vi "FGV_OEE_SQL_connection.vi"(7 "options":T4, 8 "error_in":errorcluster, 9 "all_config_info_in":T1={"main_ini_file"={"SQL Driver"="", "SQL Server"="", "SQL Database"="", "SQL UID"="", "Reference table"="", "Reference history"="", "Archivisation CFG table"="", "Archivisation CFG history"="", "User table"="", "User history"="", "Default reference"="", "Update pulse[ms]"=0, "default language"="", "SCREEN 1 Left"=10, "SCREEN 1 Top"=0, "SCREEN 1 Width"=0, "SCREEN 1 Height"=0, "SCREEN 2 Left"=0, "SCREEN 2 Top"=0, "SCREEN 2 Width"=0, "SCREEN 2 Height"=10}, "SQL Password"="", "queue_refnums"={"MAIN_queue"=refnum, "SCREEN_1_queue"=refnum, "SCREEN_2_queue"=refnum, "PULSE_queue"=refnum, "GRAPH_TOGGLE_queue"=refnum}}, 10 "SQL_transaction":string[](array[string]), 11 "SQL_statement":string) -> (0 "error_out":errorcluster, 1 "all_config_info_out":T1={"main_ini_file"={"SQL Driver"="", "SQL Server"="", "SQL Database"="", "SQL UID"="", "Reference table"="", "Reference history"="", "Archivisation CFG table"="", "Archivisation CFG history"="", "User table"="", "User history"="", "Default reference"="", "Update pulse[ms]"=0, "default language"="", "SCREEN 1 Left"=10, "SCREEN 1 Top"=0, "SCREEN 1 Width"=0, "SCREEN 1 Height"=0, "SCREEN 2 Left"=0, "SCREEN 2 Top"=0, "SCREEN 2 Width"=0, "SCREEN 2 Height"=10}, "SQL Password"="", "queue_refnums"={"MAIN_queue"=refnum, "SCREEN_1_queue"=refnum, "SCREEN_2_queue"=refnum, "PULSE_queue"=refnum, "GRAPH_TOGGLE_queue"=refnum}}, 2 "connection_active?":bool, 3 "SQL_result":variant, 4 "executed_SQL_statement":string)   [LabVIEW 2019]
uses:
  FGV_OEE_SQL_connection.ctl
  ini/typedef/OEE_all_config_info.ctl
  ini/typedef/OEE_main_ini_file.ctl
  queues/typedef/OEE_queue_refnums.ctl
  queues/typedef/OEE_MAIN_queue_element.ctl
  MAIN/OEE_MAIN_sequence_state.ctl
  queues/typedef/OEE_SCREEN_1_queue_element.ctl
  SCREEN_1/OEE_SCREEN_1_sequence_state.ctl
  queues/typedef/OEE_SCREEN_2_queue_element.ctl
  SCREEN_2/OEE_SCREEN_2_sequence_state.ctl
  queues/typedef/OEE_PULSE_queue_element.ctl
  PULSE/OEE_PULSE_sequence_state.ctl
  queues/typedef/OEE_GRAPH_TOGGLE_TIMER_queue_element.ctl
  SCREEN_2/GRAPH_TOGGLE_TIMER/OEE_GRAPH_TOGGLE_TIMER_sequence_state.ctl
  <vilib>/addons/database/Auxilliary.llb/DB Tools Transaction.ctl
  <vilib>/addons/database/Connection.llb/Conn ObjectReference.ctl
  <vilib>/addons/database/Connection.llb/DB Tools Open Connec (String).vi
  <vilib>/addons/database/Connection.llb/Conn Execute.vi
  <vilib>/addons/database/Recordset.llb/Rec Destroy - Connection.vi
  <userlib>/_OpenG.lib/array/array.llb/Filter 1D Array (String)__ogtk.vi
  <vilib>/addons/database/Recordset.llb/Rec Fetch Recordset Data (R).vi
  <vilib>/addons/database/Recordset.llb/Rec Get Recordset Properties (R).vi
  <vilib>/addons/database/Recordset.llb/Rec Get Column Properties (R).vi
  <vilib>/addons/database/Connection.llb/Conn Transaction.vi
  <vilib>/addons/database/NI_Database_API.lvlib
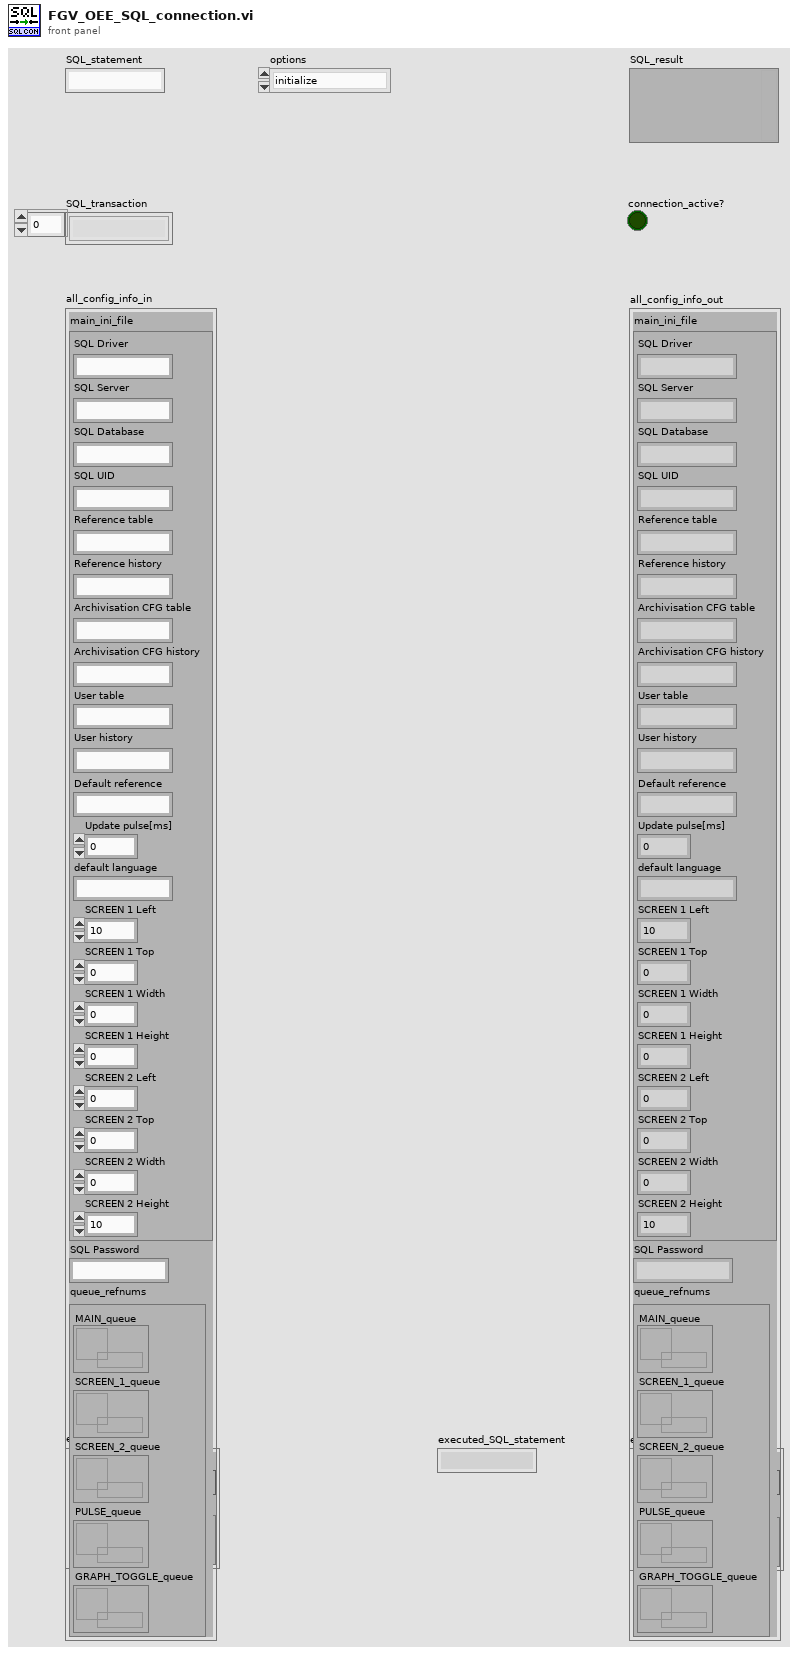
[diagram p1: front panel]
types:
  T1 = typedef "OEE_all_config_info.ctl" = cluster{"main_ini_file":T2, "SQL Password":string, "queue_refnums":T3}
  T2 = typedef "OEE_main_ini_file.ctl" = cluster{"SQL Driver":string, "SQL Server":string, "SQL Database":string, "SQL UID":string, "Reference table":string, "Reference history":string, "Archivisation CFG table":string, "Archivisation CFG history":string, "User table":string, "User history":string, "Default reference":string, "Update pulse[ms]":i32, "default language":string, "SCREEN 1 Left":i16, "SCREEN 1 Top":i16, "SCREEN 1 Width":i16, "SCREEN 1 Height":i16, "SCREEN 2 Left":i16, "SCREEN 2 Top":i16, "SCREEN 2 Width":i16, "SCREEN 2 Height":i16}
  T3 = typedef "OEE_queue_refnums.ctl" = cluster{"MAIN_queue":refnum<queue>, "SCREEN_1_queue":refnum<queue>, "SCREEN_2_queue":refnum<queue>, "PULSE_queue":refnum<queue>, "GRAPH_TOGGLE_queue":refnum<queue>}
  T4 = typedef "FGV_OEE_SQL_connection.ctl" = enum16{"initialize", "connect", "read_tables", "read_columns", "SELECT", "INSERT", "UPDATE", "DELETE", "EXEC + headers", "EXEC", "TRANSACTION", "connection_active?", "disconnect"}
  T5 = typedef "NI_Database_API.lvlib/DB Tools Transaction.ctl" = enum16{"begin", "commit", "rollback"}
  T6 = typedef "NI_Database_API.lvlib/Conn ObjectReference.ctl" = refnum<k1>
  T7 = typedef "NI_Database_API.lvlib/Rec ObjectReference.ctl" = refnum<k1>
  T8 = typedef "NI_Database_API.lvlib/Rec Properties.ctl" = cluster{"column count":i32, "record index":i32, "record count":i32, "bof?":bool, "eof?":bool, "cursor type":T9, "cache size":i32, "state":enum16{"closed", "open"}}
  T9 = typedef "NI_Database_API.lvlib/DB Tools Cursor Type.ctl" = enum16{"forward-only", "keyset", "dynamic", "static"}
  T10 = typedef "NI_Database_API.lvlib/Rec Column Properties.ctl" = cluster{"name":string, "database data type":T11, "defined size":i32, "actual size":i32}
  T11 = typedef "NI_Database_API.lvlib/DB Tools DataTypes.ctl" = enum16{"String", "Long (I32)", "Single (SGL)", "Double (DBL)", "Date/Time", "Binary"}
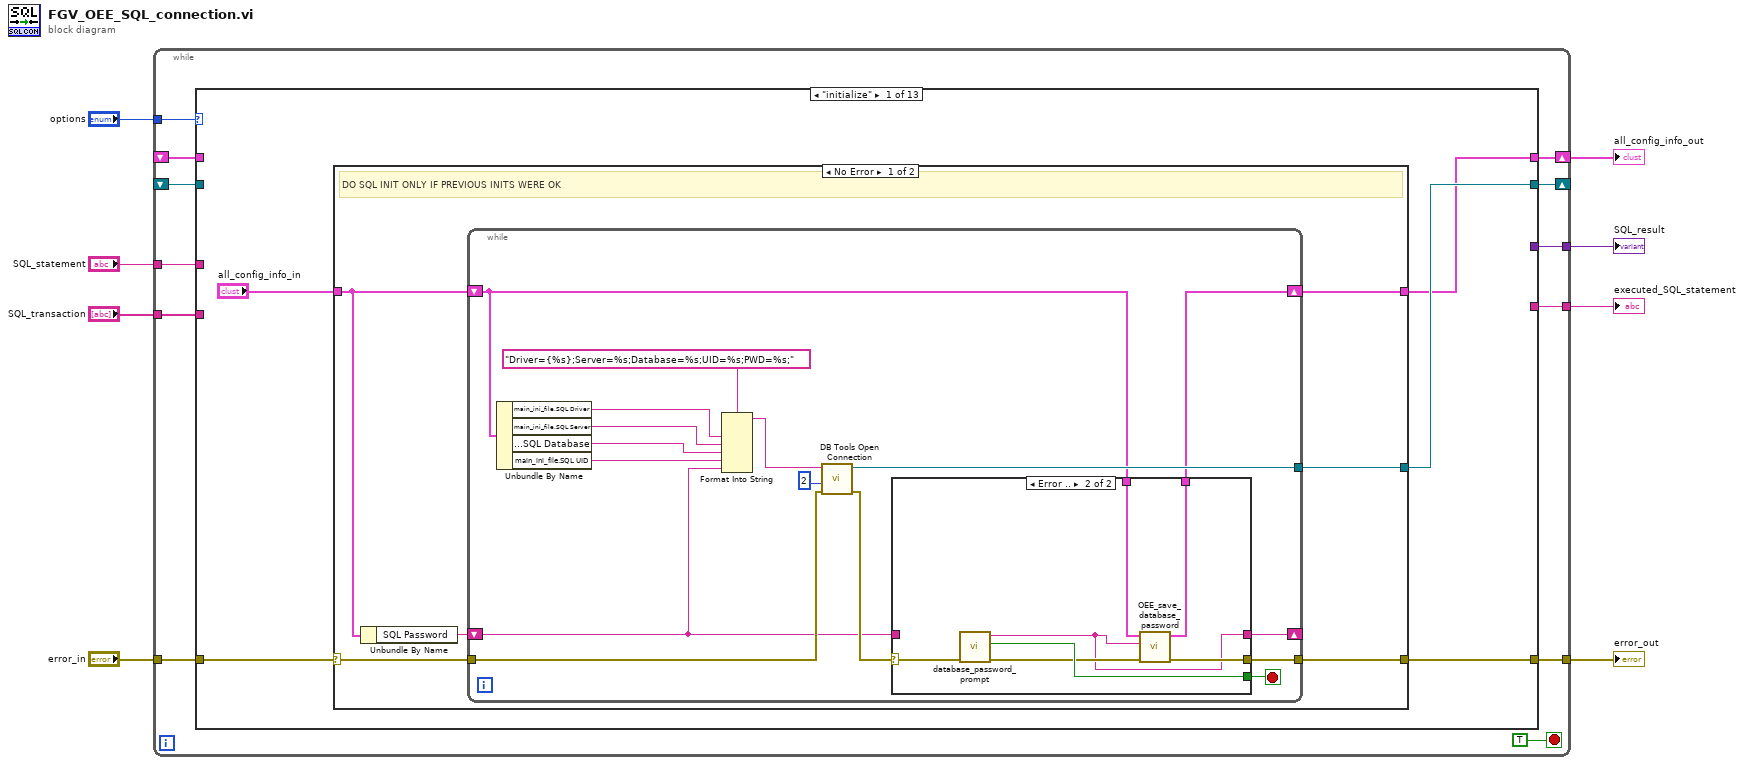
[diagram p0: block diagram]
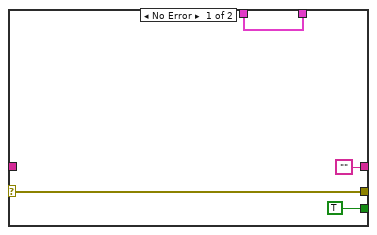
[diagram p2: hidden frame]
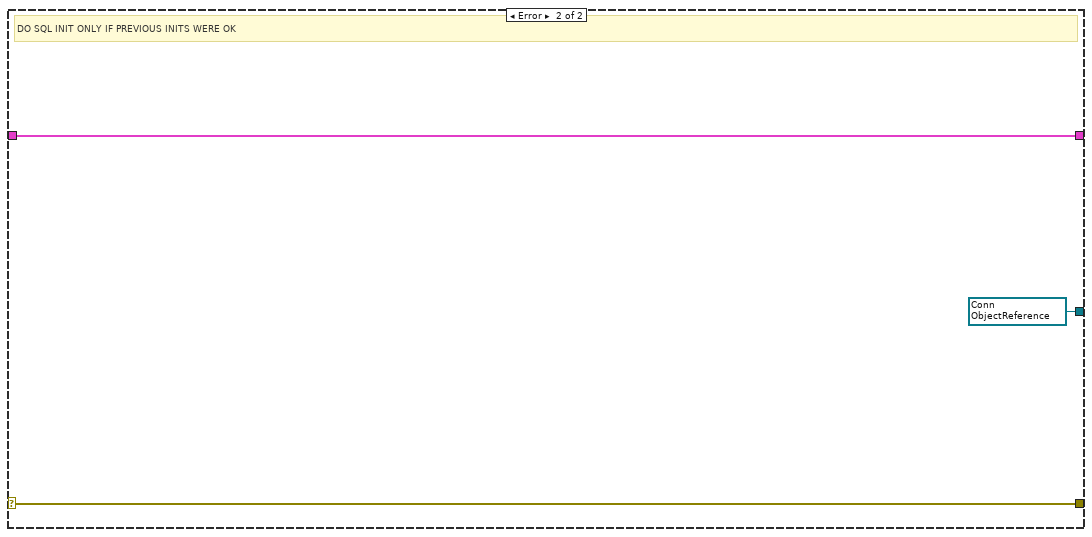
[diagram p3: hidden frame]
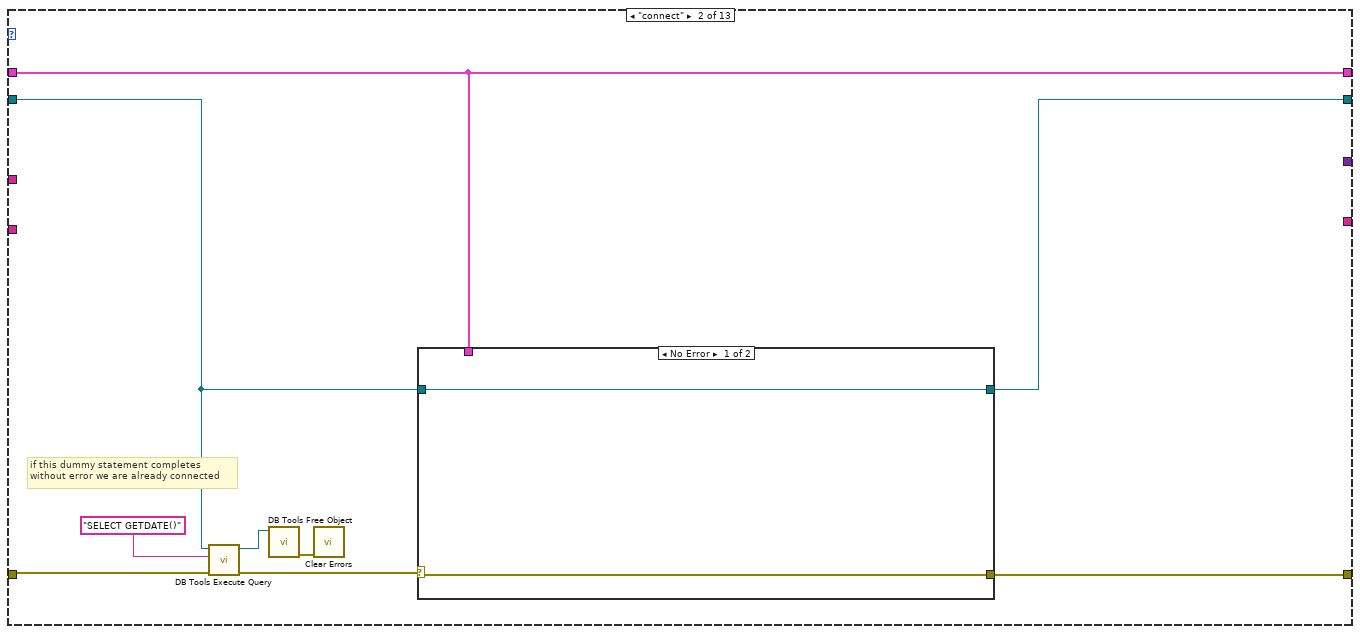
[diagram p4: hidden frame]
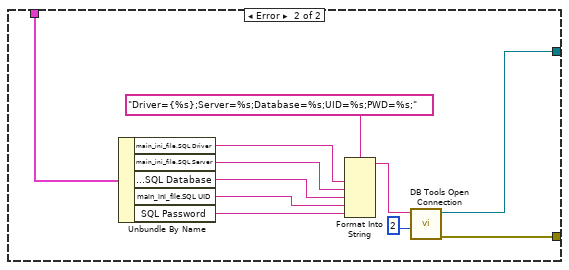
[diagram p5: hidden frame]
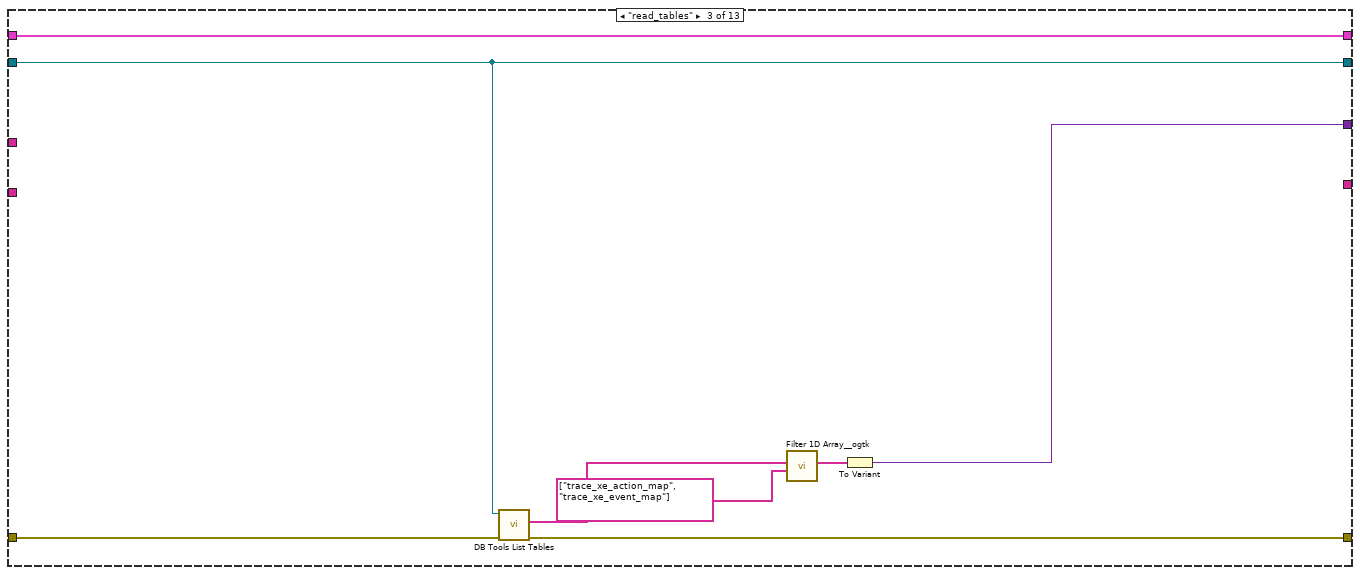
[diagram p6: hidden frame]
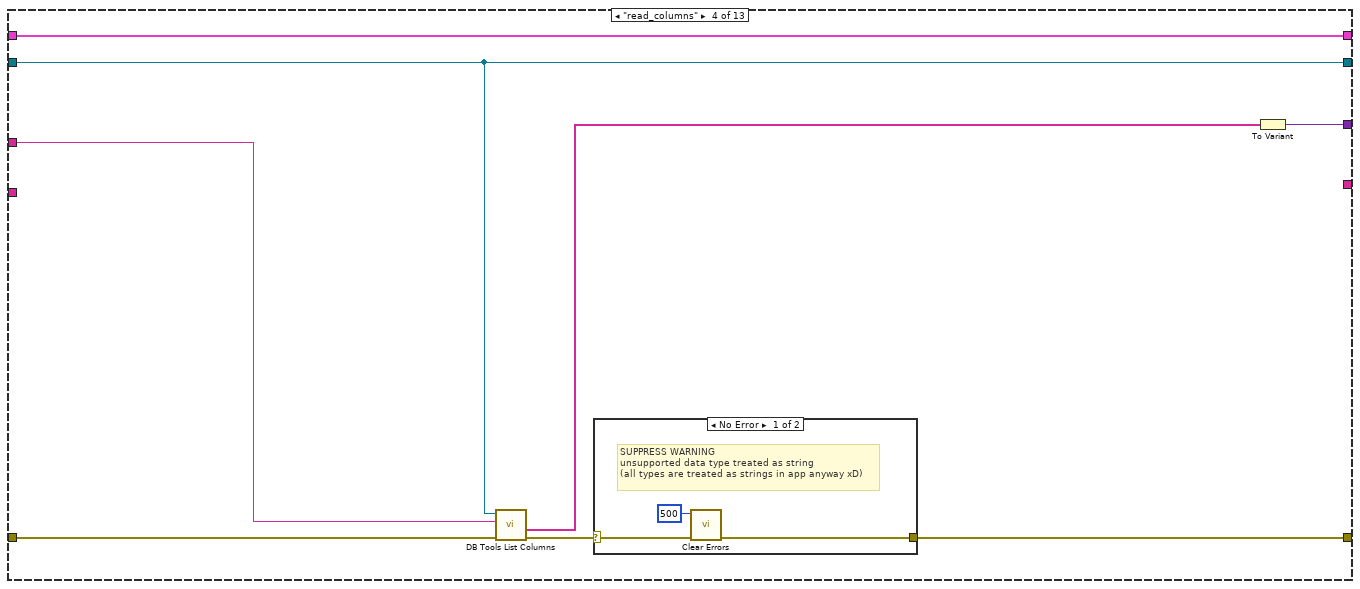
[diagram p7: hidden frame]
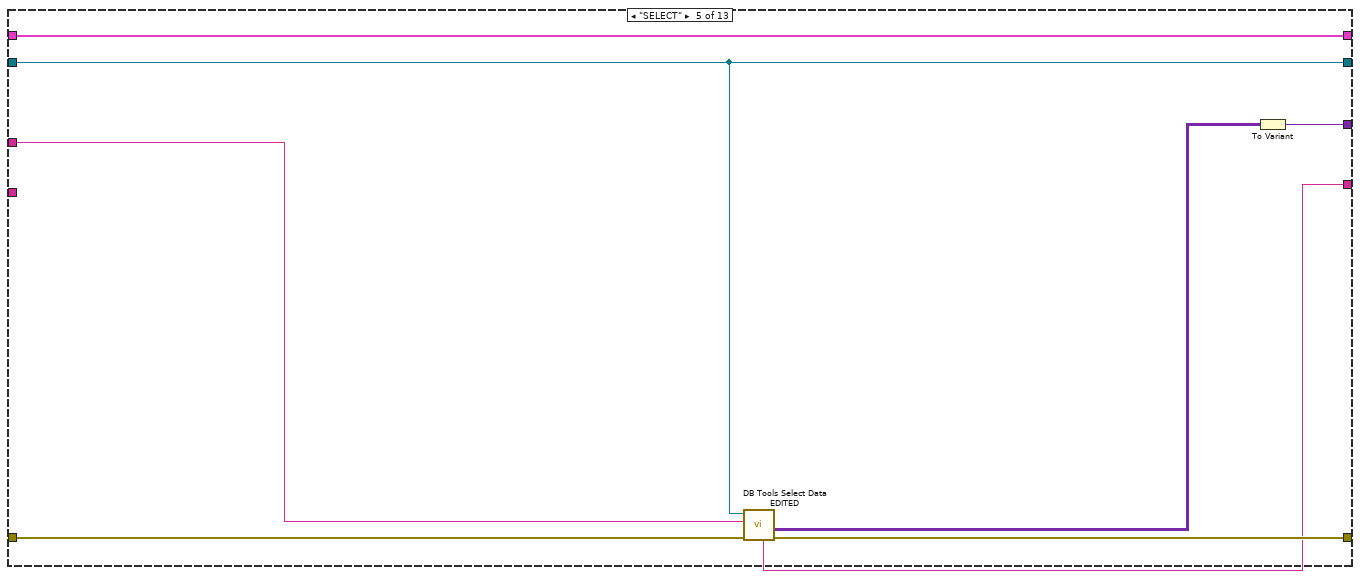
[diagram p9: hidden frame]
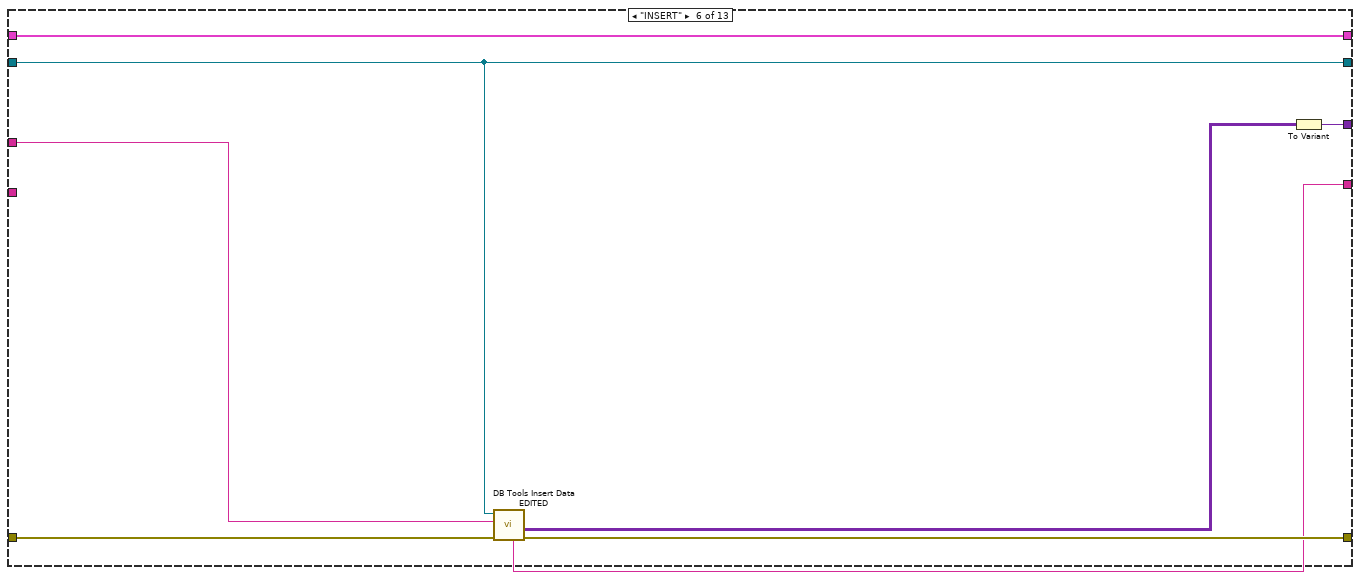
[diagram p10: hidden frame]
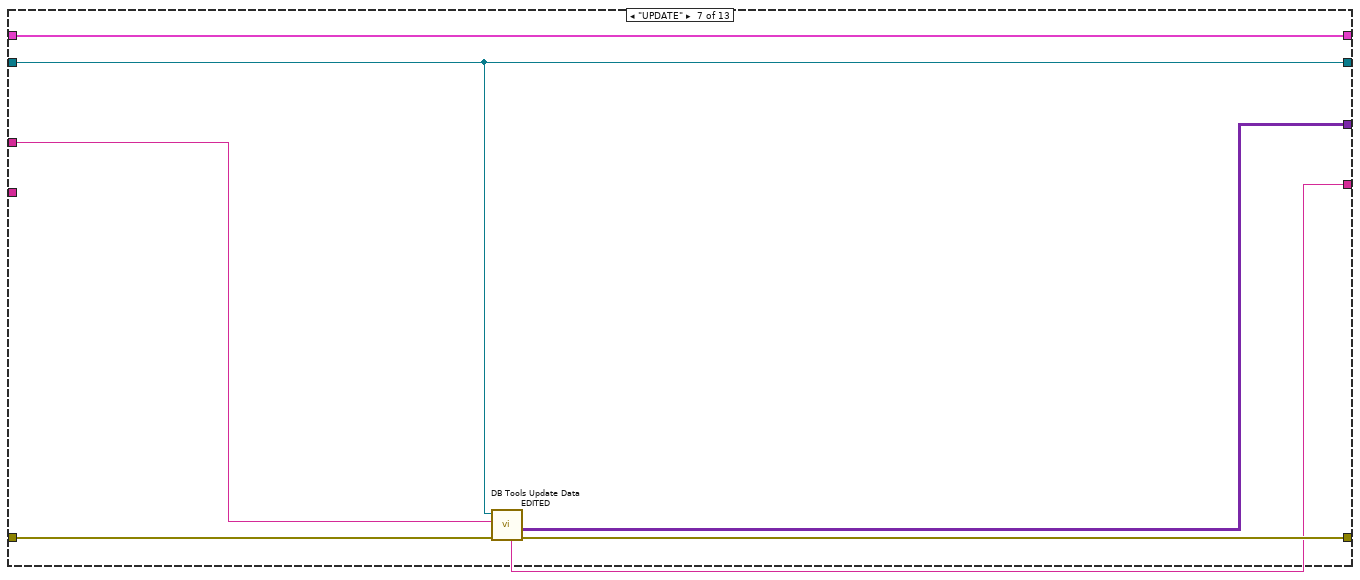
[diagram p11: hidden frame]
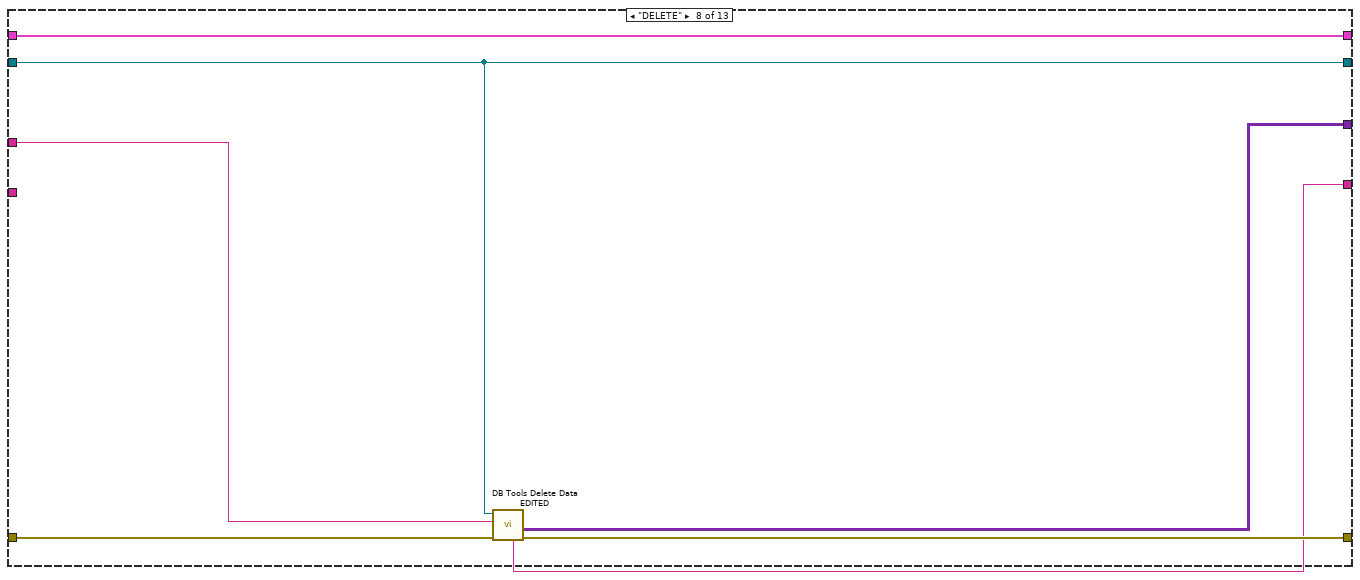
[diagram p12: hidden frame]
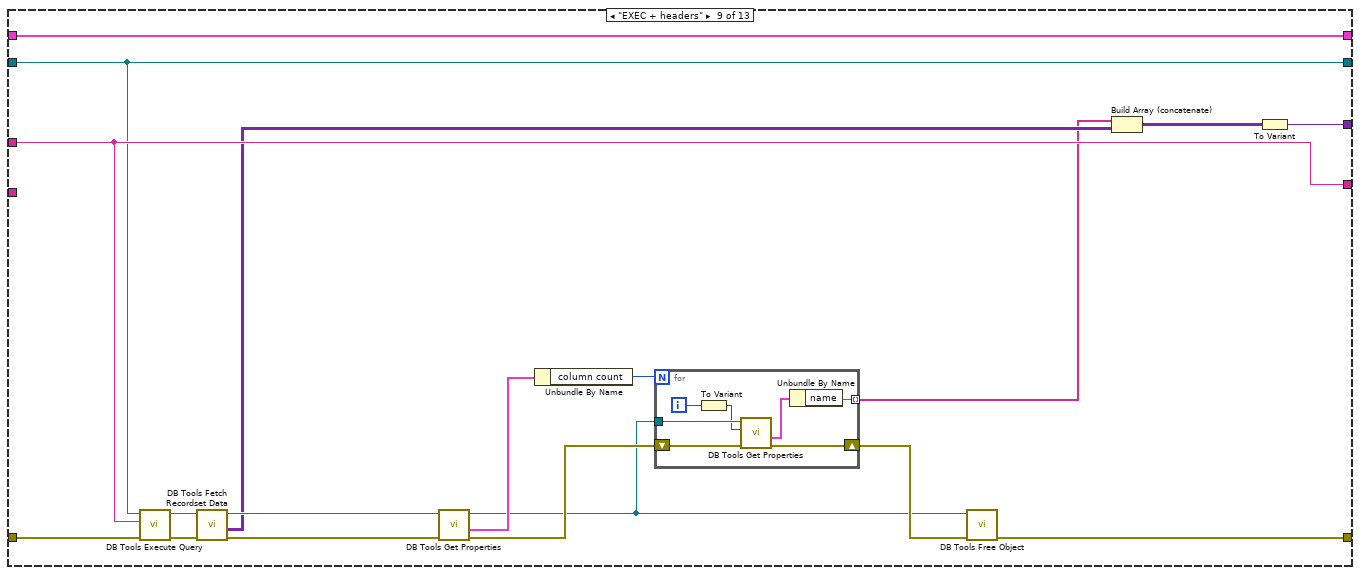
[diagram p13: hidden frame]
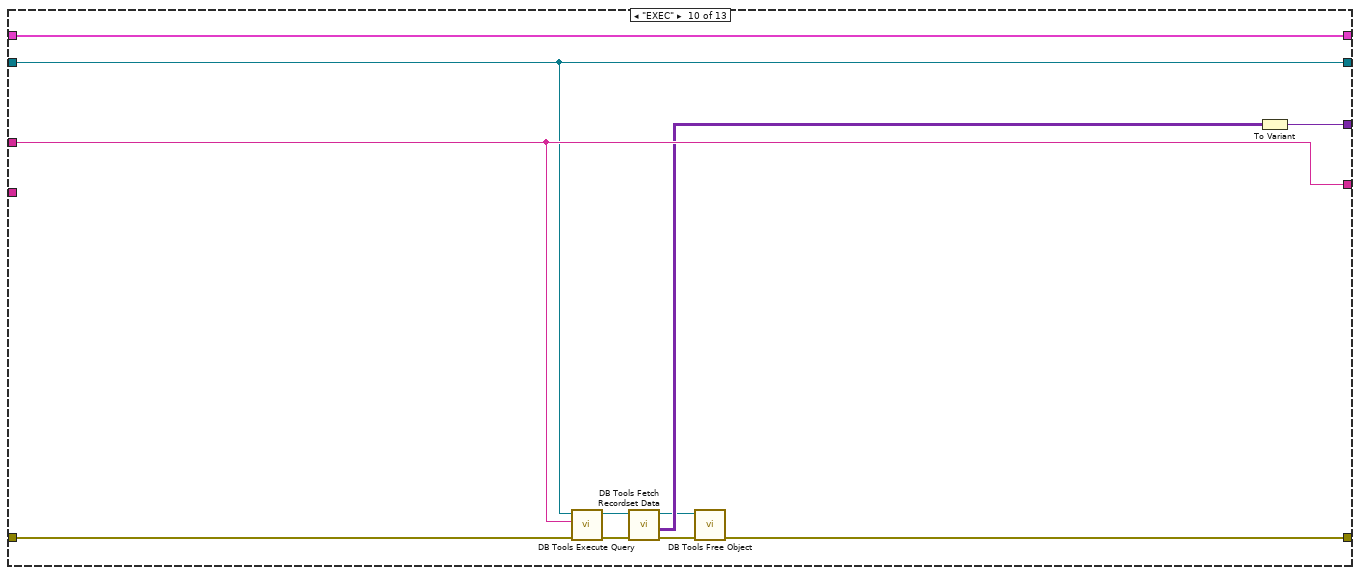
[diagram p14: hidden frame]
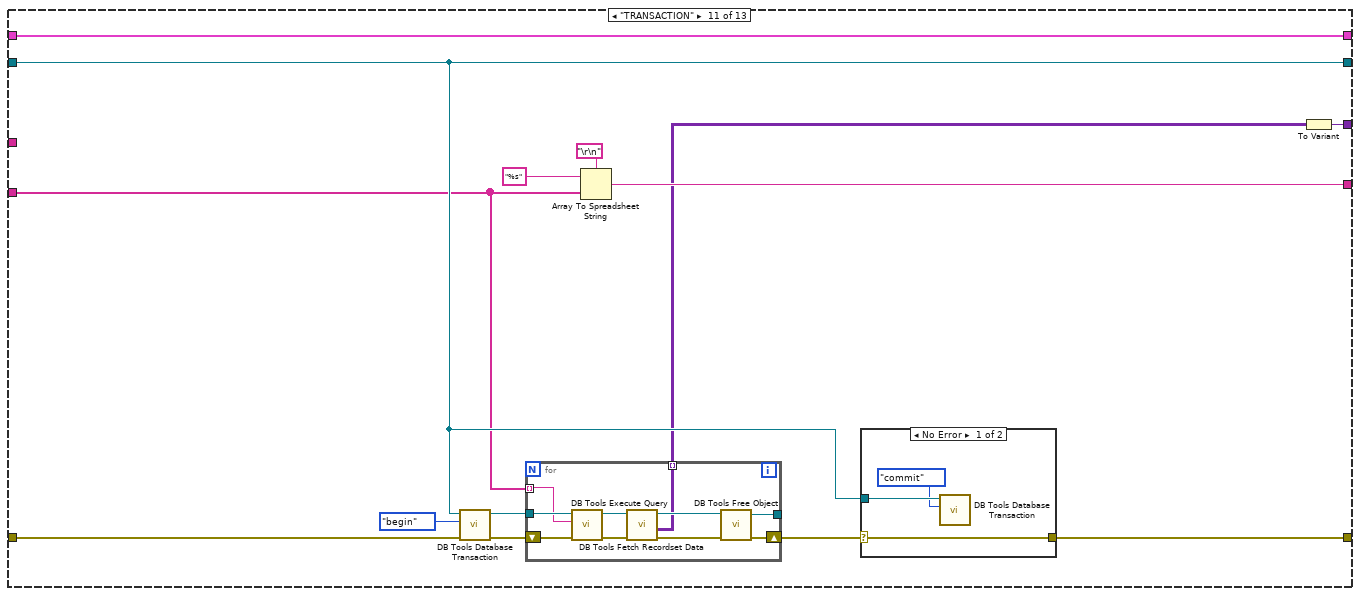
[diagram p15: hidden frame]
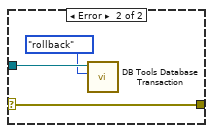
[diagram p16: hidden frame]
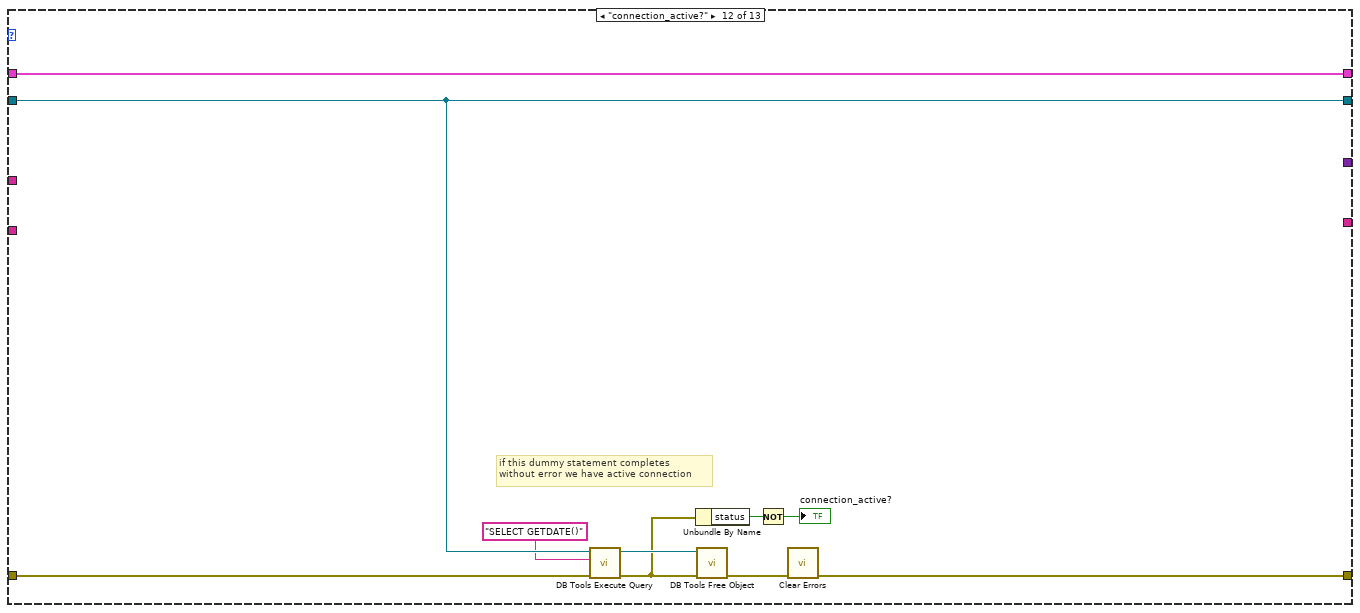
[diagram p17: hidden frame]
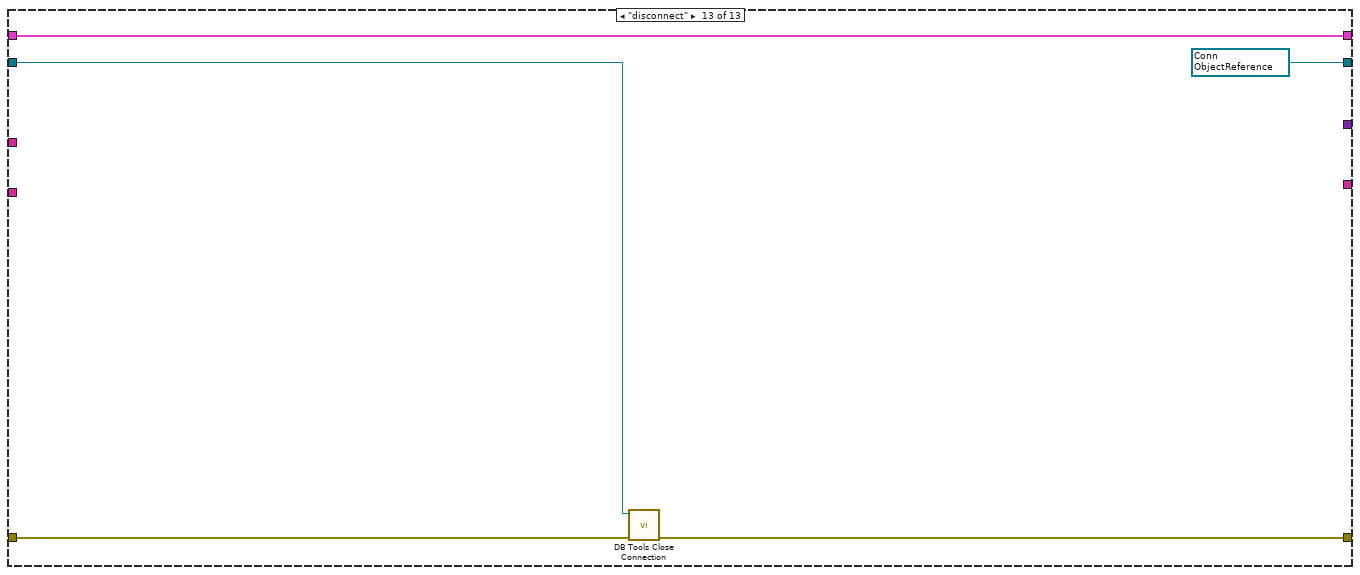
[diagram p18: hidden frame]
diagram:
  n1 = while {
    tunnel: "options" -> [w19]
    tunnel: [w18] -> w8
    tunnel: "error_in" -> [w17]
    shift-right: [w15] -> w1
    shift-left: _ -> [w16]
    shift-right: [w14] -> _
    shift-left: _ -> [w13]
    tunnel: [w12] -> w5
    tunnel: "SQL_statement" -> [w11]
    tunnel: [w10] -> w3
    tunnel: "SQL_transaction" -> [w9]
    stop <- TRUE stop-if-true
    n2 = case shown="\"initialize\"" w19 {
      tunnel: [w21 w68 w86 w92 w108 w118 w124 w132 w147 w165 w177 w205 w210] -> w18
      tunnel: w17 -> [w24 w66 w87 w98 w109 w117 w125 w131 w148 w166 w180 w209 w211]
      tunnel: w16 -> [_ w69 w91 w99 w105 w119 w126 w133 w151 w169 w183 w208 w214]
      tunnel: [w22 w69 w91 w99 w105 w119 w126 w133 w151 w169 w183 w208 w214] -> w15
      tunnel: [w25 w70 w84 w97 w110 w115 w122 w128 w145 w163 w176 w207 w212] -> w14
      tunnel: w13 -> [_ w64 w84 w97 w110 w115 w122 w128 w145 w163 w176 w207 w213]
      tunnel: [_ _ w85 w96 w111 w113 w120 w127 w144 w162 w171 _ _] -> w12
      tunnel: w11 -> [_ _ _ w94 w104 w116 w121 w129 w146 w164 _ _ _]
      tunnel: [_ _ _ _ w106 w114 w123 w130 w146 w164 w174 _ _] -> w10
      tunnel: w9 -> [_ _ _ _ _ _ _ _ _ _ w175 _ _]
      frame "initialize" {
        n3 = case shown="No Error" w24 {
          selector: w24 -> [w30 w59]
          tunnel: [w31 w61] -> w25
          tunnel: "all_config_info_in" -> [w28 w60]
          tunnel: [w26 w59] -> w21
          tunnel: [w27 w60] -> w22
          frame No Error {
            # "DO SQL INIT ONLY IF PREVIOUS INITS WERE OK"
            n4 = Unbundle By Name(w28) -> ("SQL Password"=w29:string)
            n5 = while {
              tunnel: [w42] -> w31
              shift-right: [w35] -> _
              shift-left: w29 -> [w36]
              tunnel: w30 -> [w40]
              tunnel: [w34] -> w26
              shift-right: [w33] -> w27
              shift-left: w28 -> [w32]
              stop <- w38 stop-if-true
              n6 = Unbundle By Name(w32) -> ("main_ini_file.SQL Driver"=w45:string, "main_ini_file.SQL Server"=w44:string, "main_ini_file.SQL Database"=w43:string, "main_ini_file.SQL UID"=w37:string)
              n7 = Format Into String(format string="Driver={%s};Server=%s;Database=%s;UID=%s;PWD=%s;", w45, w44, w43, w37, w36) -> (resulting string=w47:string)  [unwired: 2 in, 1 out]
              n8 = call-poly <vilib>:"DB Tools Open Connection.vi"("error in (no error)"=w40, "connection timeout (15)"=2, "connection information"=w47) -> ("error out"=w39:errorcluster, "connection reference"=w42:T6)  [unwired: 5 in]
              n9 = case shown="Error .." w39 {
                selector: w39 -> [w51 w58]
                tunnel: [w51 w53] -> w34
                tunnel: [TRUE w57] -> w38
                tunnel: w36 -> [_ _]
                tunnel: w32 -> [w49 w55]
                tunnel: [w49 w54] -> w33
                tunnel: ["" w52] -> w35
                frame No Error {
                }
                frame Error {
                  n10 = call "database_password_prompt.vi"("error_in"=w58) -> ("error_out"=w56:errorcluster, "Canceled?"=w57:bool, "new_password"=w52:string)  [unwired: 8 in]
                  n11 = call "OEE_save_database_password.vi"("error_in"=w56, "new_password"=w52, "all_config_info_in"=w55) -> ("error_out"=w53:errorcluster, "all_config_info_out"=w54:T1)  [unwired: 6 in]
                }
              }
            }
          }
          frame Error {
            w61 = T6 refnum items=["Connection"] ("connection reference")
            # "DO SQL INIT ONLY IF PREVIOUS INITS WERE OK"
          }
        }
      }
      frame "connect" {
        # "if this dummy statement completes\nwithout error we are already connected"
        n12 = call-poly <vilib>:"DB Tools Execute Query.vi"("error in (no error)"=w66, "SQL query"="SELECT GETDATE()", "connection reference"=w64) -> ("error out"=w63:errorcluster, "recordset reference"=w65:T7)  [unwired: 5 in]
        n13 = call-poly <vilib>:"DB Tools Free Object.vi"("recordset reference"=w65) -> ("error out"=w62:errorcluster)  [unwired: 9 in, 1 out]
        n14 = call <vilib>:"Clear Errors.vi"("error in (no error)"=w62) -> ()  [unwired: 5 in, 2 out]
        n15 = case shown="No Error" w63 {
          selector: w63 -> [w71 _]
          tunnel: [w72 w76] -> w70
          tunnel: w69 -> [_ w75]
          tunnel: [w71 w73] -> w68
          tunnel: w64 -> [w72 _]
          frame No Error {
          }
          frame Error {
            n16 = Unbundle By Name(w75) -> ("main_ini_file.SQL Driver"=w81:string, "main_ini_file.SQL Server"=w80:string, "main_ini_file.SQL Database"=w79:string, "main_ini_file.SQL UID"=w78:string, "SQL Password"=w77:string)
            n17 = Format Into String(format string="Driver={%s};Server=%s;Database=%s;UID=%s;PWD=%s;", w81, w80, w79, w78, w77) -> (resulting string=w83:string)  [unwired: 2 in, 1 out]
            n18 = call-poly <vilib>:"DB Tools Open Connection.vi"("connection timeout (15)"=2, "connection information"=w83) -> ("error out"=w73:errorcluster, "connection reference"=w76:T6)  [unwired: 6 in]
          }
        }
      }
      frame "read_tables" {
        n19 = call <vilib>:"DB Tools List Tables.vi"("error in (no error)"=w87, "connection reference"=w84) -> ("error out"=w86:errorcluster, "tables"=w90:string[])  [unwired: 3 in, 1 out]
        n20 = call-poly <userlib>:"Filter 1D Array__ogtk.vi"("items to filter"=string[] ["trace_xe_action_map", "trace_xe_event_map"], "array"=w90) -> ("filtered array"=w88:string[])  [unwired: 4 in, 1 out]
        n21 = To Variant(anything=w88) -> (Variant=w85:variant)
      }
      frame "read_columns" {
        n22 = call <vilib>:"DB Tools List Columns.vi"("error in (no error)"=w98, "table"=w94, "connection reference"=w97) -> ("error out"=w93:errorcluster, "columns"=w95:string[])  [unwired: 1 in, 2 out]
        n23 = case shown="No Error" w93 {
          selector: w93 -> [w102 w103]
          tunnel: [w101 w103] -> w92
          frame No Error {
            # "SUPPRESS WARNING\nunsupported data type treated as string\n(all types are treated as strings in app anyway xD)"
            n24 = call <vilib>:"Clear Errors.vi"("error in (no error)"=w102, "specific error code to clear (0: all)"=500) -> ("error out"=w101:errorcluster)  [unwired: 4 in, 1 out]
          }
          frame Error {
          }
        }
        n25 = To Variant(anything=w95) -> (Variant=w96:variant)
      }
      frame "SELECT" {
        n26 = call "DB Tools Select Data EDITED.vi"("error_in"=w109, "SELECT_statement"=w104, "connection_reference_in"=w110) -> ("error_out"=w108:errorcluster, "SQL_result"=w107:variant[][], "executed_SQL_statement"=w106:string)  [unwired: 5 in, 1 out]
        n27 = To Variant(anything=w107) -> (Variant=w111:variant)
      }
      frame "INSERT" {
        n28 = call "DB Tools Insert Data EDITED.vi"("error_in"=w117, "INSERT_statement"=w116, "connection_reference_in"=w115) -> ("error_out"=w118:errorcluster, "SQL_result"=w112:variant[][], "executed_SQL_statement"=w114:string)  [unwired: 5 in, 1 out]
        n29 = To Variant(anything=w112) -> (Variant=w113:variant)
      }
      frame "UPDATE" {
        n30 = call "DB Tools Update Data EDITED.vi"("error_in"=w125, "UPDATE_statement"=w121, "connection_reference_in"=w122) -> ("error_out"=w124:errorcluster, "SQL_result"=w120:variant[][], "executed_SQL_statement"=w123:string)  [unwired: 5 in, 1 out]
      }
      frame "DELETE" {
        n31 = call "DB Tools Delete Data EDITED.vi"("error_in"=w131, "UPDATE_statement"=w129, "connection_reference_in"=w128) -> ("error_out"=w132:errorcluster, "SQL_result"=w127:variant[][], "executed_SQL_statement"=w130:string)  [unwired: 5 in, 1 out]
      }
      frame "EXEC + headers" {
        n32 = call-poly <vilib>:"DB Tools Execute Query.vi"("error in (no error)"=w148, "SQL query"=w146, "connection reference"=w145) -> ("error out"=w150:errorcluster, "recordset reference"=w149:T7)  [unwired: 5 in]
        n33 = call-poly <vilib>:"DB Tools Fetch Recordset Data.vi"("error in (no error)"=w150, "recordset reference"=w149) -> ("error out"=w140:errorcluster, "recordset data"=w136:variant[][], "recordset reference out"=w138:T7)  [unwired: 3 in]
        n34 = call-poly <vilib>:"DB Tools Get Properties.vi"("error in (no error)"=w140, "recordset reference"=w138) -> ("error out"=w142:errorcluster, "recordset properties"=w141:T8, "recordset reference out"=w137:T7)  [unwired: 3 in]
        n35 = Unbundle By Name(w141) -> ("column count"=w143:i32)
        n36 = for {
          N: w143 -> [_]
          tunnel: w137 -> [w158]
          tunnel: [w154] -> w134 mode=indexing
          shift-right: [w152] -> w139
          shift-left: w142 -> [w153]
          i -> [w156]
          n37 = To Variant(anything=w156) -> (Variant=w157:variant)
          n38 = call-poly <vilib>:"DB Tools Get Properties.vi"("error in (no error)"=w153, "column index"=w157, "recordset reference"=w158) -> ("error out"=w152:errorcluster, "column properties"=w155:T10)  [unwired: 2 in, 1 out]
          n39 = Unbundle By Name(w155) -> ("name"=w154:string)
        }
        n40 = call-poly <vilib>:"DB Tools Free Object.vi"("error in (no error)"=w139, "recordset reference"=w137) -> ("error out"=w147:errorcluster)  [unwired: 8 in, 1 out]
        n41 = Build Array (concatenate)(w134, w136) -> (w135:variant[][])
        n42 = To Variant(anything=w135) -> (Variant=w144:variant)
      }
      frame "EXEC" {
        n43 = call-poly <vilib>:"DB Tools Execute Query.vi"("error in (no error)"=w166, "SQL query"=w164, "connection reference"=w163) -> ("error out"=w168:errorcluster, "recordset reference"=w167:T7)  [unwired: 5 in]
        n44 = call-poly <vilib>:"DB Tools Fetch Recordset Data.vi"("error in (no error)"=w168, "recordset reference"=w167) -> ("error out"=w159:errorcluster, "recordset data"=w161:variant[][], "recordset reference out"=w160:T7)  [unwired: 3 in]
        n45 = call-poly <vilib>:"DB Tools Free Object.vi"("error in (no error)"=w159, "recordset reference"=w160) -> ("error out"=w165:errorcluster)  [unwired: 8 in, 1 out]
        n46 = To Variant(anything=w161) -> (Variant=w162:variant)
      }
      frame "TRANSACTION" {
        n47 = call-poly <vilib>:"DB Tools Database Transaction.vi"("error in (no error)"=w180, "operation (begin)"=DB_Tools_Transaction."begin", "connection reference"=w176) -> ("error out"=w181:errorcluster, "connection reference out"=w179:T6)  [unwired: 3 in]
        n48 = for {
          tunnel: w179 -> [w192]
          tunnel: [w190] -> _
          shift-right: [w191] -> w178
          shift-left: w181 -> [w193]
          tunnel: w175 -> [w189] mode=indexing
          tunnel: [w184] -> w170 mode=indexing
          n49 = call-poly <vilib>:"DB Tools Execute Query.vi"("error in (no error)"=w193, "SQL query"=w189, "connection reference"=w192) -> ("error out"=w185:errorcluster, "recordset reference"=w188:T7)  [unwired: 5 in]
          n50 = call-poly <vilib>:"DB Tools Fetch Recordset Data.vi"("error in (no error)"=w185, "recordset reference"=w188) -> ("error out"=w186:errorcluster, "recordset data"=w184:variant[][], "recordset reference out"=w187:T7)  [unwired: 3 in]
          n51 = call-poly <vilib>:"DB Tools Free Object.vi"("error in (no error)"=w186, "recordset reference"=w187) -> ("error out"=w191:errorcluster, "connection reference"=w190:T6)  [unwired: 8 in]
        }
        n52 = Array To Spreadsheet String(delimiter (Tab)="\r\n", array=w175, 3:"%s" ("format string")) -> (spreadsheet string=w174:string)
        n53 = case shown="No Error" w178 {
          selector: w178 -> [w194 w197]
          tunnel: w176 -> [w196 w199]
          tunnel: [w194 w197] -> w177
          frame No Error {
            n54 = call-poly <vilib>:"DB Tools Database Transaction.vi"("operation (begin)"=DB_Tools_Transaction."commit", "connection reference"=w196) -> ()  [unwired: 4 in, 2 out]
          }
          frame Error {
            n55 = call-poly <vilib>:"DB Tools Database Transaction.vi"("operation (begin)"=DB_Tools_Transaction."rollback", "connection reference"=w199) -> ()  [unwired: 4 in, 2 out]
          }
        }
        n56 = To Variant(anything=w170) -> (Variant=w171:variant)
      }
      frame "connection_active?" {
        # "if this dummy statement completes\nwithout error we have active connection"
        n57 = call-poly <vilib>:"DB Tools Execute Query.vi"("error in (no error)"=w209, "SQL query"="SELECT GETDATE()", "connection reference"=w207) -> ("error out"=w202:errorcluster, "recordset reference"=w204:T7)  [unwired: 5 in]
        n58 = Unbundle By Name(w202) -> ("status"=w201:bool)
        n59 = call-poly <vilib>:"DB Tools Free Object.vi"("error in (no error)"=w202, "recordset reference"=w204) -> ("error out"=w203:errorcluster)  [unwired: 8 in, 1 out]
        n60 = Not(x=w201) -> (.not. x?=→"connection_active?":bool)
        n61 = call <vilib>:"Clear Errors.vi"("error in (no error)"=w203) -> ("error out"=w205:errorcluster)  [unwired: 5 in, 1 out]
      }
      frame "disconnect" {
        w212 = T6 refnum items=["Connection"] ("connection reference")
        n62 = call <vilib>:"DB Tools Close Connection.vi"("error in (no error)"=w211, "connection reference"=w213) -> ("error out"=w210:errorcluster)  [unwired: 5 in]
      }
    }
  }
  "error_out" <- w8
  "SQL_result" <- w5
  "executed_SQL_statement" <- w3
  "all_config_info_out" <- w1
